vi "terminate.vi"(8 "error in (no error)":errorcluster, 11 "GenericPlugin in":refnum<class "FPGAWrapperAN110607Galvo.lvclass">) -> (0 "error out":errorcluster, 3 "GenericPlugin out":refnum<class "FPGAWrapperAN110607Galvo.lvclass">)   [LabVIEW 2010, in "FPGAWrapperAN110607Galvo.lvclass"]
doc: "The dynamic dispatch version of this VI terminates the plug-in object by releasing all of its resources."
uses:
  FPGAWrapperAN110607Galvo.lvclass
  FPGA_VI_ref.ctl
  <vilib>/rvi/interface/nirviCloseFPGA/nirviCloseFPGA.xnode
  GenericFPGAWrapper/GenericFPGAWrapper/GenericFPGAWrapper.lvclass
  <vilib>/FPGAPlugInAG/Dynamic/niLvFpga_Close_Dynamic.vi
panel:
  in  "FPGA VI reference":T1
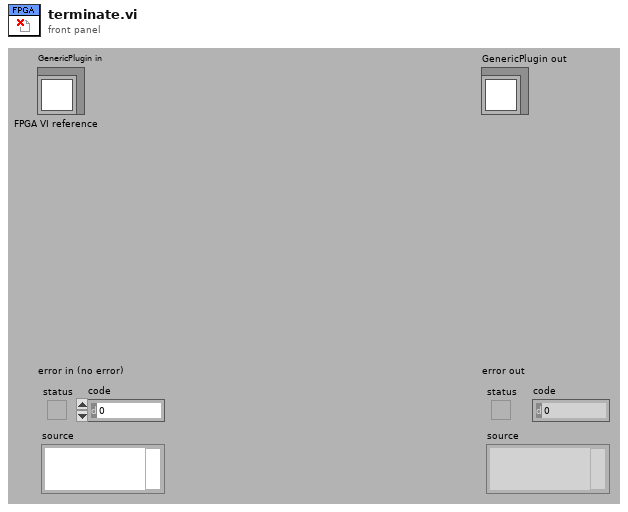
[diagram p1: front panel]
types:
  T1 = typedef "FPGAWrapperAN110607Galvo.lvclass/FPGA_VI_ref.ctl" = refnum<k20>
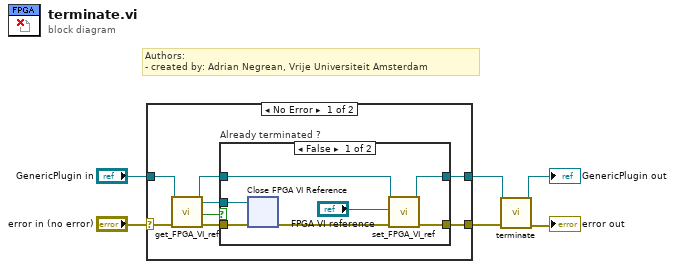
[diagram p0: block diagram]
diagram:
  # "Authors: \n- created by: Adrian Negrean, Vrije Universiteit Amsterdam"
  n1 = case shown="No Error" "error in (no error)" {
    selector: "error in (no error)" -> [w14 w30]
    tunnel: [w11 w30] -> w4
    tunnel: [w8 w31] -> w1
    tunnel: "GenericPlugin in" -> [w13 w31]
    frame No Error {
      n2 = call-dynamic "get_FPGA_VI_ref.vi"("error in (no error)"=w14, "FPGAWrapperAN110607Galvo in"=w13) -> ("error out"=w12:errorcluster, "is empty?"=w10:bool, "FPGA VI reference"=w7:T1, "FPGAWrapperAN110607Galvo out"=w9:refnum<class "FPGAWrapperAN110607Galvo.lvclass">)  [unwired: 6 in]
      n3 = case "Already terminated ?" shown="False" w10 {
        tunnel: w12 -> [w20 w29]
        tunnel: [w16 w29] -> w11
        tunnel: w9 -> [w19 w28]
        tunnel: [w18 w28] -> w8
        tunnel: w7 -> [w21 _]
        frame False {
          n4 = xnode "Close FPGA VI Reference"("FPGA VI Reference In"=w21, "error in"=w20) -> ("error out"=w17:errorcluster)
          n5 = call-dynamic "set_FPGA_VI_ref.vi"("error in (no error)"=w17, "FPGA VI reference"="FPGA VI reference", "FPGAWrapperAN110607Galvo in"=w19) -> ("error out"=w16:errorcluster, "FPGAWrapperAN110607Galvo out"=w18:refnum<class "FPGAWrapperAN110607Galvo.lvclass">)  [unwired: 7 in]
        }
        frame True {
        }
      }
    }
    frame Error {
    }
  }
  n6 = call-parent "terminate.vi"("error in (no error)"=w4, "GenericPlugin in"=w1) -> ("error out"=→"error out":errorcluster, "GenericPlugin out"=→"GenericPlugin out":refnum<class "FPGAWrapperAN110607Galvo.lvclass">)  [unwired: 8 in]
